vi "clientTest.vi"() -> ()   [LabVIEW 2011]
panel:
  in  "Lccb":string(combo)
  out "data out":string
  in  "OK Button":bool
  in  "stop":bool
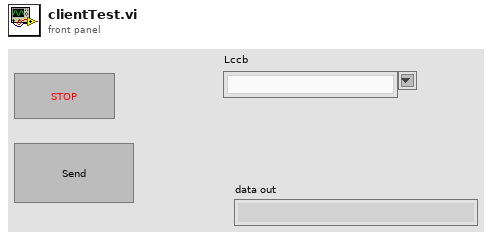
[diagram p1: front panel]
types:
  T1 = enum16{"Standard", "Buffered", "CRLF", "Immediate"}
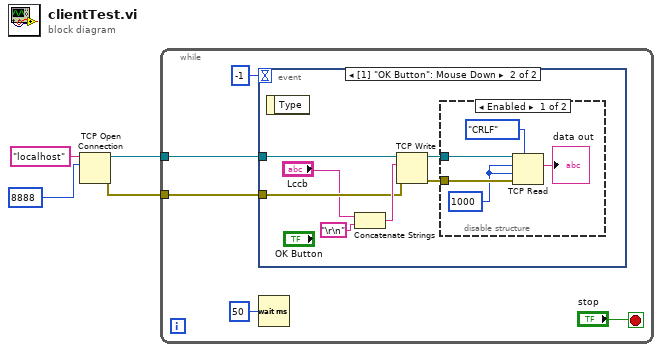
[diagram p0: block diagram]
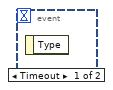
[diagram p2: hidden frame]
diagram:
  n1 = TCP Open Connection(address="localhost", remote port or service name=u16 8888) -> (connection ID=w2:refnum<k5>, error out=w1:errorcluster)  [unwired: 3 in]
  n2 = while {
    tunnel: w2 -> [w9]
    tunnel: w1 -> [w8]
    stop <- "stop" stop-if-true
    n3 = event shown="[1] \"OK Button\": Mouse Down" {
      selector: _ -> [_ _]
      dyn-events: _ -> [_ _]
      timeout: -1 -> [_ _]
      tunnel: w9 -> [_ w12]
      tunnel: w8 -> [_ w11]
      event Timeout {
        n4 = event-data() -> ()  [unwired: 1 in, 1 out]
      }
      event "OK Button": Mouse Down {
        n5 = event-data() -> ()  [unwired: 1 in, 1 out]
        n6 = Concatenate Strings("Lccb", "\r\n") -> (w15:string)
        n7 = TCP Write(connection ID=w12, data in=w15, error in (no error)=w11) -> (connection ID out=w13:refnum<k5>, error out=w14:errorcluster)  [unwired: 1 in, 1 out]
        n8 = disable-structure shown="Enabled" {
          disable-tunnel: w14 -> [w21 _]
          disable-tunnel: w13 -> [w20 _]
          frame Enabled {
            w18 = 1000 ("timeout ms (25000)")
            n9 = TCP Read(connection ID=w20, bytes to read=w18, error in (no error)=w21, 7:T1."CRLF" ("mode (standard)"), 9:w18) -> (data out=→"data out":string)  [unwired: 2 out]
          }
          frame Disabled {
          }
        }
      }
    }
    n10 = Wait (ms)(milliseconds to wait=u32 50) -> ()  [unwired: 1 out]
  }
